vi "Bead Comp Calculation (SubVI).vi"(10 "Bead In":cluster{dbl[], dbl[]}, 11 "Gain Parameters":T1={"For Every (mm)"=0.1, "Override by (%)"=6.0, "Deadband (%)"=4.0, "Saturation H (%)"=100.0, "Saturation L (%)"=100.0}) -> (3 "Compensation Out (%)":cluster{dbl[], dbl[]})   [LabVIEW 2016]
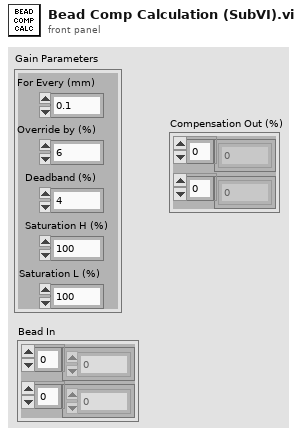
[diagram p1: front panel]
types:
  T1 = cluster{"For Every (mm)":dbl, "Override by (%)":dbl, "Deadband (%)":dbl, "Saturation H (%)":dbl, "Saturation L (%)":dbl}
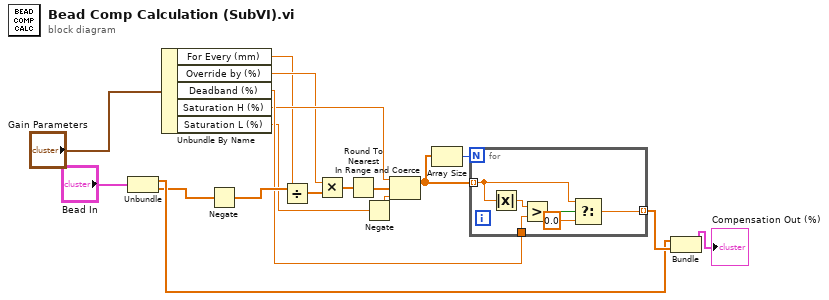
[diagram p0: block diagram]
diagram:
  n1 = Unbundle("Bead In") -> (w15:dbl[], w5:dbl[])
  n2 = Unbundle By Name("Gain Parameters") -> ("For Every (mm)"=w4:dbl, "Override by (%)"=w7:dbl, "Deadband (%)"=w14:dbl, "Saturation H (%)"=w10:dbl, "Saturation L (%)"=w1:dbl)
  n3 = Negate(x=w5) -> (-x=w18:dbl[])
  n4 = Divide(x=w18, y=w4) -> (x/y=w6:dbl[])
  n5 = Multiply(x=w7, y=w6) -> (x*y=w8:dbl[])
  n6 = Round To Nearest(number=w8) -> (nearest integer value=w9:dbl[])
  n7 = Negate(x=w1) -> (-x=w11:dbl)
  n8 = In Range and Coerce(upper limit=w10, x=w9, lower limit=w11) -> (coerced(x)=w13:dbl[])  [unwired: 1 out]
  n9 = Array Size(array=w13) -> (size(s)=w12:i32)
  n10 = for {
    N: w12 -> [_]
    tunnel: w13 -> [w21] mode=indexing
    tunnel: w14 -> [w22]
    tunnel: [w19] -> w16 mode=indexing
    n11 = Absolute Value(x=w21) -> (abs(x)=w23:dbl)
    n12 = Greater?(x=w23, y=w22) -> (0:w24:bool)
    n13 = Select(t=w21, s=w24, f=0.0) -> (s? t:f=w19:dbl)
  }
  n14 = Bundle(w15, w16) -> (→"Compensation Out (%)":cluster{dbl[], dbl[]})  [unwired: 1 in]
